vi "VI Tree - numeric__ogtk.vi"   [LabVIEW 2018]
uses:
  <userlib>/_OpenG.lib/numeric/numeric.llb/Random Number Within Range - DBL__ogtk.vi
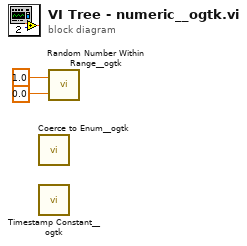
[diagram p0: block diagram]
diagram:
  n1 = call <userlib>:"Coerce to Enum__ogtk.vi"() -> ()  [unwired: 1 in]
  n2 = call <userlib>:"Timestamp Constant__ogtk.vi"() -> ()  [unwired: 1 in]
  n3 = call-poly <userlib>:"Random Number Within Range__ogtk.vi"("High"=1.0 ("High (1.00)"), "Low"=0.0 ("Low (0.00)")) -> ()  [unwired: 3 in, 1 out]
